vi "limit_pct.vi"(5 "upper limit":dbl=1.0, 7 "lower limit":dbl=-1.0, 11 "PCT":dbl) -> (3 "PCT Out":dbl)   [LabVIEW 2015]
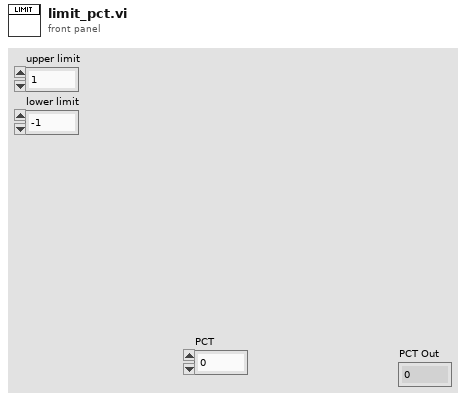
[diagram p1: front panel]
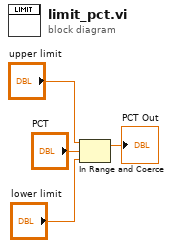
[diagram p0: block diagram]
diagram:
  n1 = In Range and Coerce(upper limit="upper limit", x="PCT", lower limit="lower limit") -> (coerced(x)=→"PCT Out":dbl)  [unwired: 1 out]
